vi "Read Command Sequence File.vi"(11 "Path Name":string) -> (3 "Auto Commands":T1[](array[typedef]))   [LabVIEW 2019]
uses:
  Controls/Auto Controls.ctl
  <vilib>/Utility/file.llb/Read Delimited Spreadsheet (DBL).vi
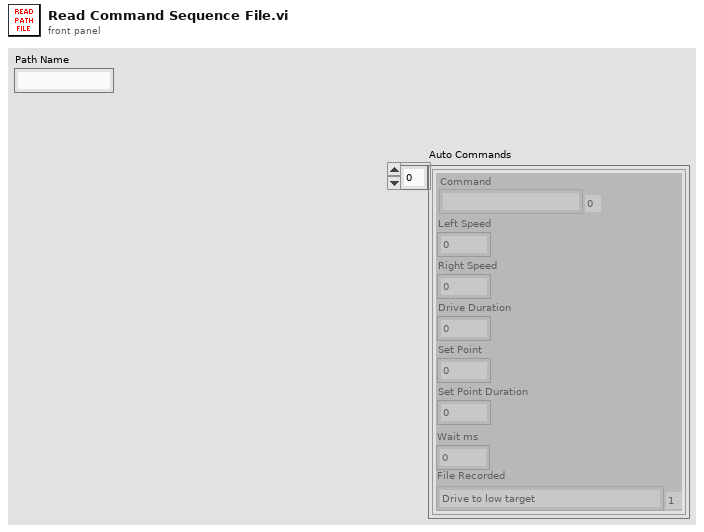
[diagram p1: front panel]
types:
  T1 = typedef "Auto Controls.ctl" = cluster{"Drive Duration":dbl, "Left Speed":dbl, "Right Speed":dbl, "Set Point":dbl, "Set Point Duration":dbl, "Command":enum16{"", "Drive Forwards", "Drive Backwards", "Stop", "Turn Left", "Turn Right", "Drop Intake", "Lift Intake", "Intake", "Shooter", "Transfer", "Wait", "Drive from recorded file"}, "Wait ms":dbl, "File Recorded":enum16{"None", "Drive to low target", "Drive to pick balls from the right CP", "Drive to pick up balls from the Left CP", "Drive to pick up 3 balls from the center", "Drive to pick up 2 balls from the center"}}
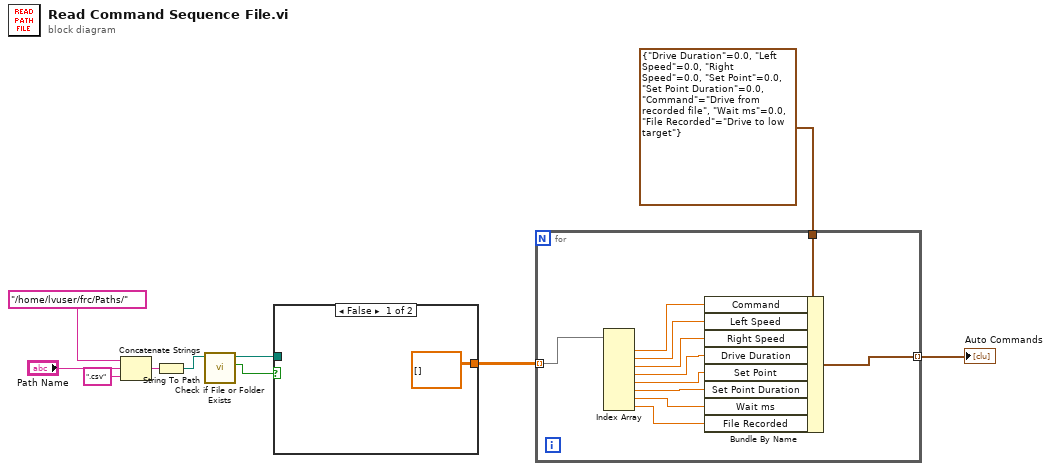
[diagram p0: block diagram]
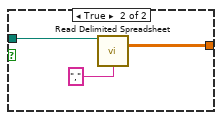
[diagram p2: hidden frame]
diagram:
  n1 = Concatenate Strings("/home/lvuser/frc/Paths/" ("string"), "Path Name", ".csv" ("string")) -> (w5:string)
  n2 = String To Path(string=w5) -> (path=w4:path)
  n3 = call <vilib>:"Check if File or Folder Exists.vi"("path"=w4) -> ("file or folder exists?"=w8:bool, "dup path"=w7:path)  [unwired: 8 in, 1 out]
  n4 = case shown="False" w8 {
    tunnel: w7 -> [_ w14]
    tunnel: [dbl[][] [] ("all rows") w12] -> w1
    frame False {
    }
    frame True {
      n5 = call-poly <vilib>:"Read Delimited Spreadsheet.vi"("file path (dialog if empty)"=w14, "delimiter (\\t)"="," ("delimiter (\\t)")) -> ("all rows"=w12:dbl[][])  [unwired: 8 in, 5 out]
    }
  }
  n6 = for {
    tunnel: T1 {"Drive Duration"=0.0, "Left Speed"=0.0, "Right Speed"=0.0, "Set Point"=0.0, "Set Point Duration"=0.0, "Command"=enum."Drive from recorded file", "Wait ms"=0.0, "File Recorded"=enum."Drive to low target"} ("Auto Control") -> [w25]
    tunnel: [w17] -> w3 mode=indexing
    tunnel: w1 -> [w16] mode=indexing
    n7 = Index Array(array=w16) -> (element #1=w24:dbl, element #2=w23:dbl, element #3=w22:dbl, element #4=w21:dbl, element #5=w20:dbl, element #6=w19:dbl, element #7=w18:dbl, element #8=w15:dbl)  [unwired: 8 in]
    n8 = Bundle By Name(cluster=w25, "Command"=w24, "Left Speed"=w23, "Right Speed"=w22, "Drive Duration"=w21, "Set Point"=w20, "Set Point Duration"=w19, "Wait ms"=w18, "File Recorded"=w15) -> (w17:T1)
  }
  "Auto Commands" <- w3
